vi "Show ADC Readings.vi"() -> ()   [LabVIEW 2012]
uses:
  Type/_RT Command.ctl
  Type/_RT Configuration 2.ctl
  <vilib>/Utility/config.llb/Read Key (I32).vi
  <vilib>/Utility/config.llb/Read Key (String).vi
  Configuration/_Global Configuration.vi
  <vilib>/Utility/config.llb/Write Key (I32).vi
  <vilib>/Utility/config.llb/Write Key (String).vi
  <vilib>/Utility/config.llb/NI_LVConfig.lvlib
panel:
  in  "Export":bool
  in  "Import":bool
  in  "Reserved":sgl=1.0
  in  "Tolerance":sgl
  out "Bit Pattern":i16 format="%012b"
  in  "Read":bool
  in  "Slope":sgl=1.0
  in  "Offset":sgl
  in  "Channel Name":string="Q1-ADC1-1"
  in  "Listbox":i32(listbox)
  # "(MSB)"
  # "(Enter a new value to make changes to the current row)"
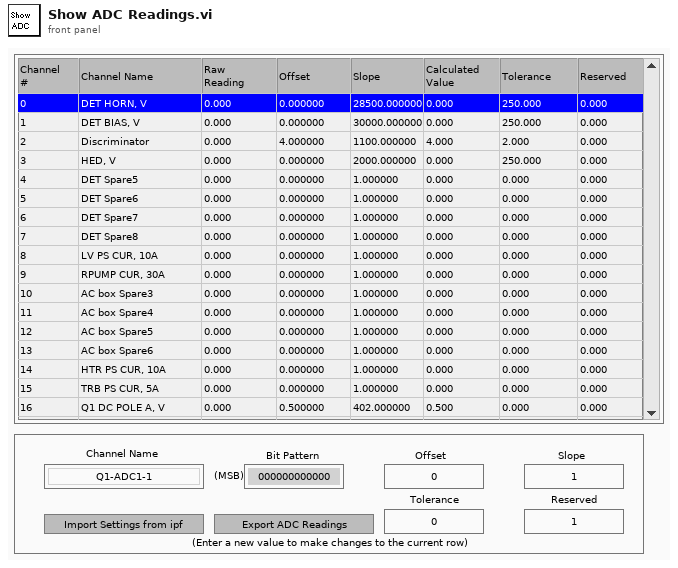
[diagram p1: front panel]
types:
  T1 = typedef "_RT Command.ctl" = enum16{"Start", "Stop", "Runtime Update", "Get Data", "Get Info", "Get Status", "Get Param", "Get Config", "Get Table", "Read ADC", "Set Oscillator", "Update Config", "Update Table", "Set All Pol", "Set Pol and DC", "Set Max Mass", "Toggle RP", "Toggle EL", "Set PIC", "Initialize Turbo", "Send Turbo Comm", "Close Turbo", "P1", "P2", "P3", "Send Serial", "Set LC Out", "Get LC In", "Read VAC", "Test Table", "Toggle Power", "Get Startup", "Set Startup", "Get ADC Table", "Set ADC Table", "Get Brief Status", "Get Detail Status", "Auxiliary Update", "Set CC Logics", "Set CC Input Logics", "Ignore Error"}
  T2 = enum32{"existing file", "new file", "new or existing file", "existing dir", "new dir", "new or existing dir", "existing file (use LLBs)", "new file (use LLBs)", "new or existing file (use LLBs)", "new or existing file or directory (use LLBs)"}
  T3 = typedef "_RT Configuration 2.ctl" = cluster{"Name":string, "Ch#":u8, "Min":dbl, "Max":dbl, "Def+":dbl, "Def-":dbl, "Offset":dbl, "Slope":dbl, "Type":u8, "Description":string, "SettleT":dbl}
  T4 = typedef "NI_LVConfig.lvlib/Config Data RefNum.ctl" = refnum<k1>
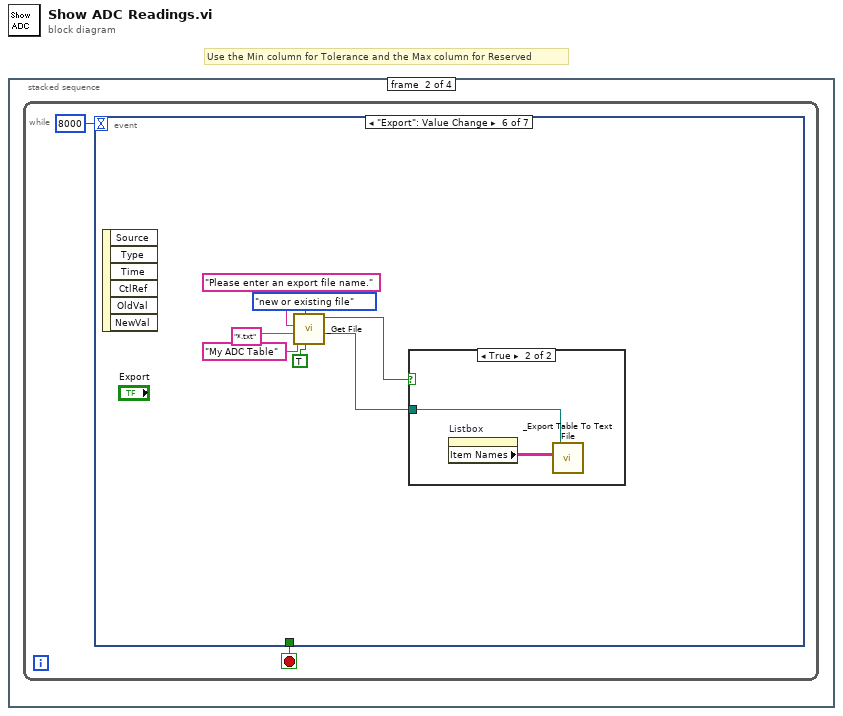
[diagram p0: block diagram]
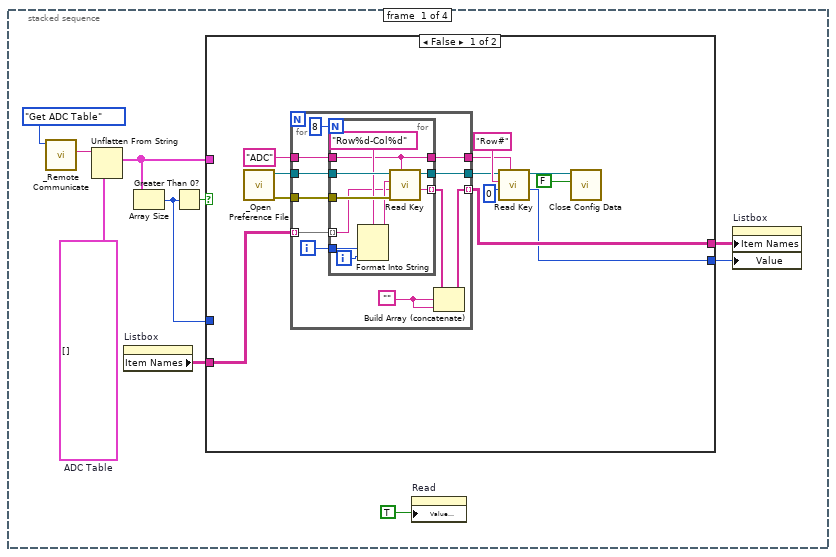
[diagram p2: hidden frame]
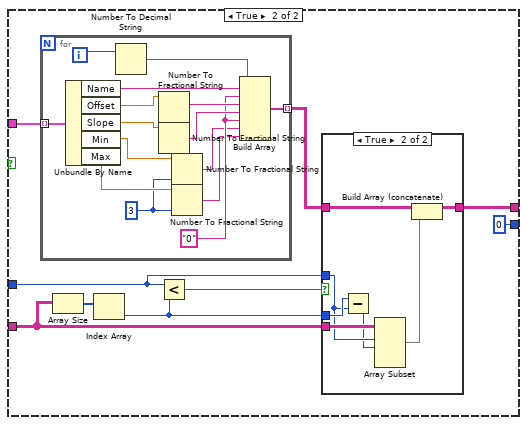
[diagram p3: hidden frame]
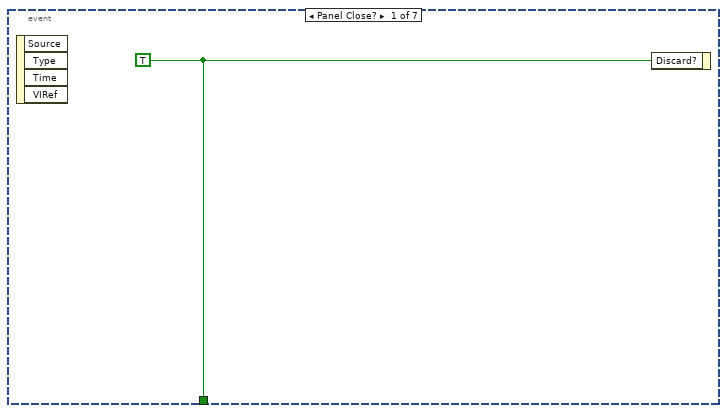
[diagram p5: hidden frame]
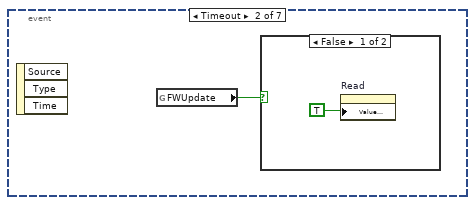
[diagram p6: hidden frame]
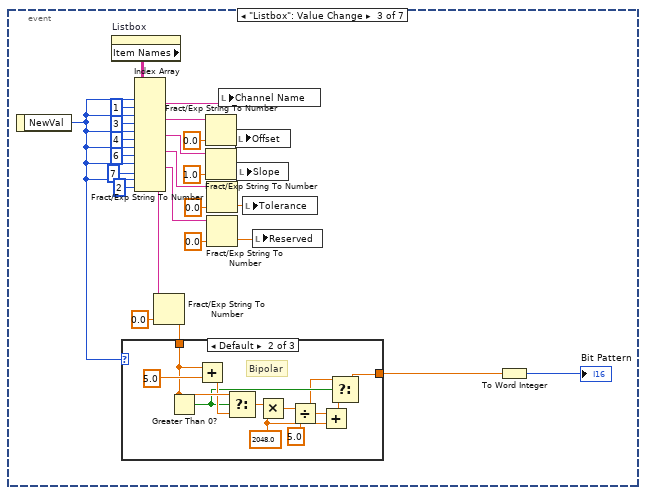
[diagram p8: hidden frame]
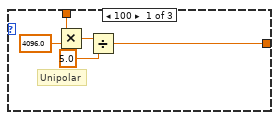
[diagram p9: hidden frame]
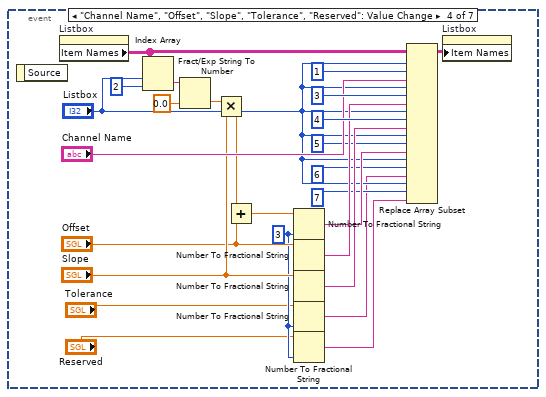
[diagram p11: hidden frame]
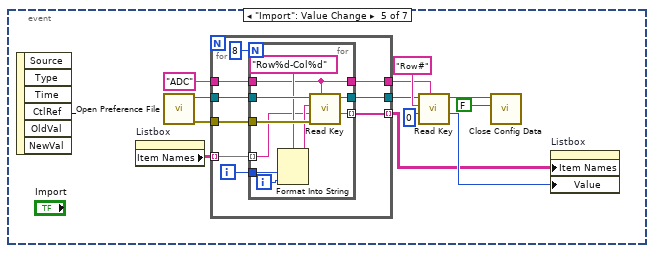
[diagram p12: hidden frame]
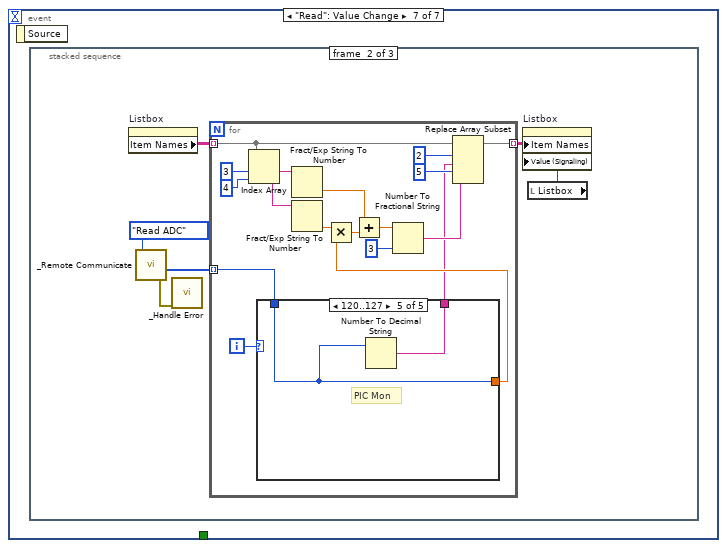
[diagram p14: hidden frame]
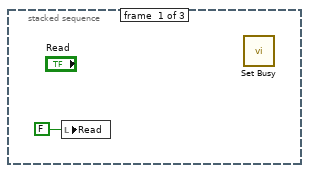
[diagram p15: hidden frame]
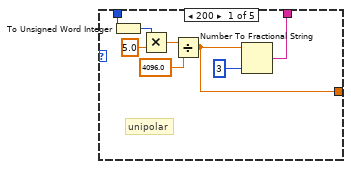
[diagram p16: hidden frame]
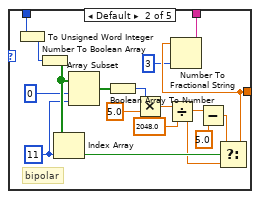
[diagram p17: hidden frame]
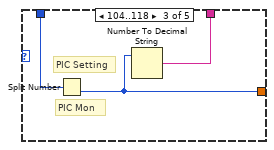
[diagram p18: hidden frame]
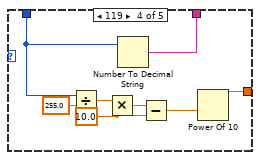
[diagram p19: hidden frame]
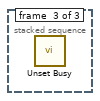
[diagram p20: hidden frame]
diagram:
  # "Use the Min column for Tolerance and the Max column for Reserved"
  n1 = stacked-sequence {
    frame #0 {
      w3 = T3[] []  # ADC Table
      n2 = call "_Remote Communicate.vi"("Command"=_RT_Command."Get ADC Table") -> ("Info"=w6:string)  [unwired: 5 in, 3 out]
      n3 = Unflatten From String(type=w3, binary string=w6) -> (value=w4:T3[])  [unwired: 1 in, 4 out]
      n4 = property on="Listbox" class="MCListbox (strict)"() -> ("Item Names"=w2:string[][])  [unwired: 2 in, 2 out]
      n5 = Array Size(array=w4) -> (size(s)=w1:i32)
      n6 = Greater Than 0?(x=w1) -> (x > 0?=w5:bool)
      n7 = case shown="False" w5 {
        tunnel: [w17 w45] -> w9
        tunnel: [w12 0 ("value")] -> w8
        tunnel: w4 -> [_ w51]
        tunnel: w2 -> [w11 w50]
        tunnel: w1 -> [_ w47]
        frame False {
          n8 = call "_Open Preference File.vi"() -> ("error"=w15:errorcluster, "refnum"=w16:T4)  [unwired: 1 in, 5 out]
          n9 = for {
            tunnel: w16 -> [w33]
            tunnel: w15 -> [w32]
            tunnel: "ADC" ("section") -> [w31]
            tunnel: [w29] -> w18
            tunnel: w11 -> [w27] mode=indexing
            tunnel: [w23] -> w17 mode=indexing
            tunnel: [w26] -> w19
            i -> [w28]
            w25 = ""
            n10 = for {
              N: 8 -> [_]
              tunnel: w33 -> [w43]
              tunnel: w32 -> [w42]
              tunnel: w31 -> [w34]
              tunnel: [w41] -> w29
              tunnel: w28 -> [w39]
              tunnel: w27 -> [w36] mode=indexing
              tunnel: [w35] -> w24 mode=indexing
              tunnel: [w34] -> w26
              i -> [w40]
              n11 = Format Into String(format string="Row%d-Col%d" ("section"), w39, w40) -> (resulting string=w37:string)  [unwired: 2 in, 1 out]
              n12 = call-poly <vilib>:"Read Key.vi"("section"=w34, "error in (no error)"=w42, "default value"=w36, "key"=w37, "refnum"=w43) -> ("value"=w35:string, "refnum out"=w41:T4)  [unwired: 1 in, 4 out]
            }
            n13 = Build Array (concatenate)(w24, w25, w25) -> (w23:string[])
          }
          n14 = call-poly <vilib>:"Read Key.vi"("section"=w19, "default value"=0 ("Listbox"), "key"="Row#" ("section"), "refnum"=w18) -> ("value"=w12:i32, "refnum out"=w21:T4)  [unwired: 1 in, 5 out]
          n15 = call <vilib>:"Close Config Data.vi"("write file if changed (T)"=FALSE ("write configuration file? (T)"), "refnum"=w21) -> ()  [unwired: 1 in, 9 out]
        }
        frame True {
          n16 = for {
            tunnel: w51 -> [w75] mode=indexing
            tunnel: [w61] -> w44 mode=indexing
            i -> [w74]
            w64 = "0"
            w69 = i16 3 ("precision (6)")
            n17 = Unbundle By Name(w75) -> ("Name"=w67:string, "Offset"=w73:dbl, "Slope"=w72:dbl, "Min"=w71:dbl, "Max"=w70:dbl)
            n18 = Number To Decimal String(number=w74) -> (decimal integer string=w68:string)  [unwired: 1 out]
            n19 = Number To Fractional String(number=w73) -> (F-format string=w66:string)  [unwired: 3 out]
            n20 = Number To Fractional String(number=w72) -> (F-format string=w65:string)  [unwired: 3 out]
            n21 = Number To Fractional String(number=w71, precision (6)=w69) -> (F-format string=w63:string)  [unwired: 2 out]
            n22 = Number To Fractional String(number=w70, precision (6)=w69) -> (F-format string=w62:string)  [unwired: 2 out]
            n23 = Build Array(w68, w67, w64, w66, w65, w64, w63, w62) -> (w61:string[])
          }
          n24 = Array Size(array=w50) -> (size(s)=w49:i32[])
          n25 = Index Array(array=w49) -> (element=w46:i32)  [unwired: 1 in]
          n26 = Less?(x=w47, y=w46) -> (x < y?=w48:bool)
          n27 = case shown="True" w48 {
            tunnel: w50 -> [_ w59]
            tunnel: w47 -> [_ w58]
            tunnel: w46 -> [_ w60]
            tunnel: w44 -> [w53 w56]
            tunnel: [w53 w55] -> w45
            frame False {
            }
            frame True {
              n28 = Subtract(x=w60, y=w58) -> (x-y=w57:i32)
              n29 = Array Subset(array=w59, index (row)=w58, length (row)=w57) -> (w54:string[][])  [unwired: 2 in]
              n30 = Build Array (concatenate)(w56, w54) -> (w55:string[][])
            }
          }
        }
      }
      n31 = property on="Read" class="Bool (strict)"("Value (Signaling)"=TRUE) -> ()  [unwired: 2 in, 2 out]
      n32 = property on="Listbox" class="MCListbox (strict)"("Item Names"=w9, "Value"=w8) -> ()  [unwired: 2 in, 2 out]
    }
    frame #1 {
      n33 = while {
        stop <- w77 stop-if-true
        n34 = event shown="[5] \"Export\": Value Change" {
          selector: _ -> [_ _ _ _ _ _ _]
          dyn-events: _ -> [_ _ _ _ _ _ _]
          timeout: 8000 -> [_ _ _ _ _ _ _]
          tunnel: [w78 _ _ _ _ _ _] -> w77
          event Panel Close? {
            w78 = TRUE ("Discard?")
            n35 = event-data() -> ()  [unwired: 5 out]
            n36 = event-data("Discard?"=w78) -> ()  [unwired: 1 in, 1 out]
          }
          event Timeout {
            n37 = event-data() -> ()  [unwired: 4 out]
            n38 = global read "_Global Configuration.vi" "FWUpdate"() -> (w79:bool)
            n39 = case shown="False" w79 {
              frame False {
                n40 = property on="Read" class="Bool (strict)"("Value (Signaling)"=TRUE) -> ()  [unwired: 2 in, 2 out]
              }
              frame True {
              }
            }
          }
          event "Listbox": Value Change {
            n41 = event-data() -> ("NewVal"=w89:i32)  [unwired: 1 out]
            n42 = property on="Listbox" class="MCListbox (strict)"() -> ("Item Names"=w106:string[][])  [unwired: 2 in, 2 out]
            n43 = Index Array(array=w106, index (row) #1=w89, index (col) #1=1 ("disabled index (col)"), index (row) #2=w89, index (col) #2=3 ("disabled index (col)"), index (row) #3=w89, index (col) #3=4 ("disabled index (col)"), index (row) #4=w89, index (col) #4=6 ("disabled index (col)"), index (row) #5=w89, index (col) #5=7 ("disabled index (col)"), index (row) #6=w89, index (col) #6=2 ("index (col)")) -> (element #1=w100:string, element #2=w102:string, element #3=w101:string, element #4=w83:string, element #5=w82:string, element #6=w81:string)
            n44 = Fract/Exp String To Number(string=w81, default (0 dbl)=sgl 0.0 ("default (0 DBL)")) -> (number=w93:sgl)  [unwired: 3 out]
            n45 = case shown="Default" w89 {
              tunnel: w93 -> [w111 w119 w123]
              tunnel: [w107 w113 w123] -> w92
              frame 100 {
                # "Unipolar"
                n46 = Multiply(x=w111, y=sgl 4096.0) -> (x*y=w109:sgl)
                n47 = Divide(x=w109, y=sgl 5.0) -> (x/y=w107:sgl)
              }
              frame Default {
                w112 = sgl 2048.0 ("y")
                # "Bipolar"
                n48 = Greater Than 0?(x=w119) -> (x > 0?=w116:bool)
                n49 = Add(x=w119, y=sgl 5.0) -> (x+y=w118:sgl)
                n50 = Select(t=w119, s=w116, f=w118) -> (s? t:f=w117:sgl)
                n51 = Multiply(x=w117, y=w112) -> (x*y=w122:sgl)
                n52 = Divide(x=w122, y=sgl 5.0) -> (x/y=w115:sgl)
                n53 = Add(x=w115, y=w112) -> (x+y=w114:sgl)
                n54 = Select(t=w115, s=w116, f=w114) -> (s? t:f=w113:sgl)
              }
              frame 104..127 {
              }
            }
            n55 = Fract/Exp String To Number(string=w102, default (0 dbl)=sgl 0.0 ("default (0 DBL)")) -> (number=w99:sgl)  [unwired: 3 out]
            n56 = Fract/Exp String To Number(string=w101, default (0 dbl)=sgl 1.0 ("default (0 DBL)")) -> (number=w97:sgl)  [unwired: 3 out]
            n57 = Fract/Exp String To Number(string=w83, default (0 dbl)=sgl 0.0 ("default (0 DBL)")) -> (number=w84:sgl)  [unwired: 3 out]
            n58 = Fract/Exp String To Number(string=w82, default (0 dbl)=sgl 0.0 ("default (0 DBL)")) -> (number=w86:sgl)  [unwired: 3 out]
            n59 = local write "Channel Name"(w100) -> ()
            n60 = local write "Offset"(w99) -> ()
            n61 = local write "Slope"(w97) -> ()
            n62 = local write "Tolerance"(w84) -> ()
            n63 = local write "Reserved"(w86) -> ()
            n64 = To Word Integer(number=w92) -> (16bit integer=→"Bit Pattern":i16)
          }
          event "Channel Name", "Offset", "Slope", "Tolerance", "Reserved": Value Change {
            w131 = i16 3 ("precision (6)")
            n65 = event-data() -> ()  [unwired: 2 out]
            n66 = property on="Listbox" class="MCListbox (strict)"() -> ("Item Names"=w141:string[][])  [unwired: 2 in, 2 out]
            n67 = Index Array(array=w141, index (row)="Listbox", index (col)=2 ("disabled index (col)")) -> (element=w139:string)
            n68 = Fract/Exp String To Number(string=w139, default (0 dbl)=sgl 0.0 ("default (0 DBL)")) -> (number=w137:sgl)  [unwired: 3 out]
            n69 = Multiply(x=w137, y="Slope") -> (x*y=w135:sgl)
            n70 = Add(x=w135, y="Offset") -> (x+y=w133:sgl)
            n71 = Number To Fractional String(number=w133, precision (6)=w131) -> (F-format string=w132:string)  [unwired: 2 out]
            n72 = Number To Fractional String(number="Offset") -> (F-format string=w144:string)  [unwired: 3 out]
            n73 = Number To Fractional String(number="Slope") -> (F-format string=w143:string)  [unwired: 3 out]
            n74 = Number To Fractional String(number="Tolerance", precision (6)=w131) -> (F-format string=w125:string)  [unwired: 2 out]
            n75 = Number To Fractional String(number="Reserved", precision (6)=w131) -> (F-format string=w124:string)  [unwired: 2 out]
            n76 = Replace Array Subset(array=w141, new element #1="Channel Name", index (row) #1="Listbox", index (col) #1=1 ("disabled index (col)"), new element #2=w144, index (row) #2="Listbox", index (col) #2=3 ("disabled index (col)"), new element #3=w143, index (row) #3="Listbox", index (col) #3=4 ("disabled index (col)"), new element #4=w132, index (row) #4="Listbox", index (col) #4=5 ("disabled index (col)"), new element #5=w125, index (row) #5="Listbox", index (col) #5=6 ("disabled index (col)"), new element #6=w124, index (row) #6="Listbox", index (col) #6=7 ("disabled index (col)")) -> (w146:string[][])
            n77 = property on="Listbox" class="MCListbox (strict)"("Item Names"=w146) -> ()  [unwired: 2 in, 2 out]
          }
          event "Import": Value Change {
            n78 = event-data() -> ()  [unwired: 7 out]
            n79 = property on="Listbox" class="MCListbox (strict)"() -> ("Item Names"=w151:string[][])  [unwired: 2 in, 2 out]
            n80 = call "_Open Preference File.vi"() -> ("error"=w153:errorcluster, "refnum"=w154:T4)  [unwired: 1 in, 5 out]
            n81 = for {
              tunnel: w154 -> [w170]
              tunnel: w153 -> [w169]
              tunnel: "ADC" ("section") -> [w168]
              tunnel: [w166] -> w155
              tunnel: w151 -> [w163] mode=indexing
              tunnel: [w162] -> w160 mode=indexing
              tunnel: [w164] -> w156
              i -> [w165]
              n82 = for {
                N: 8 -> [_]
                tunnel: w170 -> [w180]
                tunnel: w169 -> [w179]
                tunnel: w168 -> [w171]
                tunnel: [w178] -> w166
                tunnel: w165 -> [w176]
                tunnel: w163 -> [w173] mode=indexing
                tunnel: [w172] -> w162 mode=indexing
                tunnel: [w171] -> w164
                i -> [w177]
                n83 = Format Into String(format string="Row%d-Col%d" ("section"), w176, w177) -> (resulting string=w174:string)  [unwired: 2 in, 1 out]
                n84 = call-poly <vilib>:"Read Key.vi"("section"=w171, "error in (no error)"=w179, "default value"=w173, "key"=w174, "refnum"=w180) -> ("value"=w172:string, "refnum out"=w178:T4)  [unwired: 1 in, 4 out]
              }
            }
            n85 = call-poly <vilib>:"Read Key.vi"("section"=w156, "default value"=0 ("Listbox"), "key"="Row#" ("section"), "refnum"=w155) -> ("value"=w161:i32, "refnum out"=w158:T4)  [unwired: 1 in, 5 out]
            n86 = call <vilib>:"Close Config Data.vi"("write file if changed (T)"=FALSE ("write configuration file? (T)"), "refnum"=w158) -> ()  [unwired: 1 in, 9 out]
            n87 = property on="Listbox" class="MCListbox (strict)"("Item Names"=w160, "Value"=w161) -> ()  [unwired: 2 in, 2 out]
          }
          event "Export": Value Change {
            n88 = event-data() -> ()  [unwired: 7 out]
            n89 = call "_Get File.vi"("For Write (T)"=TRUE, "select mode (new or existing)"=T2."new or existing file", "default name"="My ADC Table", "extension (isd)"="*.txt" ("pattern (all files)"), "prompt"="Please enter an export file name.") -> ("Seleted File"=w181:path, "Succeeded"=w182:bool)  [unwired: 1 in, 2 out]
            n90 = case shown="True" w182 {
              tunnel: w181 -> [_ w188]
              frame False {
              }
              frame True {
                n91 = property on="Listbox" class="MCListbox (strict)"() -> ("Item Names"=w189:string[][])  [unwired: 2 in, 2 out]
                n92 = call "_Export Table To Text File.vi"("2D data"=w189, "file path (dialog if empty)"=w188) -> ()  [unwired: 4 in, 3 out]
              }
            }
          }
          event "Read": Value Change {
            n93 = event-data() -> ()  [unwired: 2 out]
            n94 = stacked-sequence {
              frame #0 {
                n95 = local write "Read"(FALSE ("Undo")) -> ()
                n96 = call <vilib>:"Set Busy.vi"() -> ()  [unwired: 4 in, 8 out]
              }
              frame #1 {
                n97 = property on="Listbox" class="MCListbox (strict)"() -> ("Item Names"=w194:string[][])  [unwired: 2 in, 2 out]
                n98 = call "_Remote Communicate.vi"("Command"=_RT_Command."Read ADC") -> ("error out"=w192:errorcluster, "Data Array"=w191:i32[])  [unwired: 5 in, 2 out]
                n99 = call "_Handle Error.vi"("error in (no error)"=w192) -> ()  [unwired: 2 in, 5 out]
                n100 = for {
                  tunnel: [w203] -> w196 mode=indexing
                  tunnel: w191 -> [w198] mode=indexing
                  tunnel: w194 -> [w202] mode=indexing
                  i -> [w201]
                  n101 = Index Array(array=w202, index #1=3 ("index"), index #2=4 ("index")) -> (element #1=w212:string, element #2=w211:string)
                  n102 = case shown="120..127" w201 {
                    tunnel: [w218 w225 w240 w243 w251] -> w200
                    tunnel: w198 -> [w216 w228 w242 w244 w251]
                    tunnel: [w217 w223 w241 w245 w252] -> w197
                    frame 200 {
                      # "unipolar"
                      n103 = To Unsigned Word Integer(number=w216) -> (unsigned 16bit integer=w215:u16)
                      n104 = Multiply(x=w215, y=sgl 5.0) -> (x*y=w221:sgl)
                      n105 = Divide(x=w221, y=sgl 4096.0) -> (x/y=w218:sgl)
                      n106 = Number To Fractional String(number=w218, precision (6)=i16 3) -> (F-format string=w217:string)  [unwired: 2 out]
                    }
                    frame Default {
                      w237 = 11 ("index")
                      # "bipolar"
                      n107 = To Unsigned Word Integer(number=w228) -> (unsigned 16bit integer=w227:u16)
                      n108 = Number To Boolean Array(number=w227) -> (Boolean array=w239:bool[])
                      n109 = Index Array(array=w239, index=w237) -> (element=w232:bool)
                      n110 = Array Subset(array=w239, index=0, length=w237) -> (w236:bool[])
                      n111 = Boolean Array To Number(Boolean array=w236) -> (number=w233:u32)
                      n112 = Multiply(x=w233, y=sgl 5.0) -> (x*y=w226:sgl)
                      n113 = Divide(x=w226, y=sgl 2048.0) -> (x/y=w231:sgl)
                      n114 = Subtract(x=w231, y=sgl 5.0) -> (x-y=w229:sgl)
                      n115 = Select(t=w229, s=w232, f=w231) -> (s? t:f=w225:sgl)
                      n116 = Number To Fractional String(number=w225, precision (6)=i16 3) -> (F-format string=w223:string)  [unwired: 2 out]
                    }
                    frame 104..118 {
                      # "PIC Setting"
                      # "PIC Mon"
                      n117 = Split Number(x=w242) -> (lo(x)=w240:u16)  [unwired: 1 out]
                      n118 = Number To Decimal String(number=w240) -> (decimal integer string=w241:string)  [unwired: 1 out]
                    }
                    frame 119 {
                      w246 = sgl 10.0 ("y")
                      n119 = Divide(x=w244, y=sgl 255.0) -> (x/y=w249:sgl)
                      n120 = Multiply(x=w249, y=w246) -> (x*y=w248:sgl)
                      n121 = Number To Decimal String(number=w244) -> (decimal integer string=w245:string)  [unwired: 1 out]
                      n122 = Subtract(x=w248, y=w246) -> (x-y=w247:sgl)
                      n123 = Power Of 10(x=w247) -> (10^x=w243:sgl)
                    }
                    frame 120..127 {
                      # "PIC Mon"
                      n124 = Number To Decimal String(number=w251) -> (decimal integer string=w252:string)  [unwired: 1 out]
                    }
                  }
                  n125 = Fract/Exp String To Number(string=w212) -> (number=w208:dbl)  [unwired: 4 out]
                  n126 = Fract/Exp String To Number(string=w211) -> (number=w210:dbl)  [unwired: 4 out]
                  n127 = Multiply(x=w210, y=w200) -> (x*y=w209:dbl)
                  n128 = Add(x=w208, y=w209) -> (x+y=w207:dbl)
                  n129 = Number To Fractional String(number=w207, precision (6)=i16 3) -> (F-format string=w199:string)  [unwired: 2 out]
                  n130 = Replace Array Subset(array=w202, new element #1=w197, index #1=2 ("index"), new element #2=w199, index #2=5 ("index")) -> (w203:string[])
                }
                n131 = local read "Listbox"() -> (w195:i32)
                n132 = property on="Listbox" class="MCListbox (strict)"("Item Names"=w196, "Value (Signaling)"=w195) -> ()  [unwired: 2 in, 2 out]
              }
              frame #2 {
                n133 = call <vilib>:"Unset Busy.vi"() -> ()  [unwired: 2 in, 10 out]
              }
            }
          }
        }
      }
    }
    frame #2 {
      n134 = property on="Listbox" class="MCListbox (strict)"() -> ("Item Names"=w257:string[][])  [unwired: 2 in, 2 out]
      n135 = call "_Open Preference File.vi"() -> ("error"=w266:errorcluster, "refnum"=w267:T4)  [unwired: 1 in, 5 out]
      n136 = for {
        tunnel: w267 -> [w288]
        tunnel: "ADC" ("section") -> [w286]
        tunnel: [w284] -> w264
        tunnel: w257 -> [w282] mode=indexing
        tunnel: [w281] -> w262
        shift-right: [w280] -> w259
        shift-left: w266 -> [w287]
        i -> [w283]
        n137 = for {
          N: 8 -> [_]
          tunnel: w288 -> [w298]
          tunnel: w286 -> [w290]
          tunnel: [w296] -> w284
          tunnel: w283 -> [w294]
          tunnel: w282 -> [w291] mode=indexing
          tunnel: [w290] -> w281
          shift-right: [w289] -> w280
          shift-left: w287 -> [w297]
          i -> [w295]
          n138 = Format Into String(format string="Row%d-Col%d" ("section"), w294, w295) -> (resulting string=w292:string)  [unwired: 2 in, 1 out]
          n139 = call-poly <vilib>:"Write Key.vi"("section"=w290, "error in (no error)"=w297, "value"=w291, "key"=w292, "refnum"=w298) -> ("error out"=w289:errorcluster, "refnum out"=w296:T4)  [unwired: 1 in, 4 out]
        }
      }
      n140 = for {
        tunnel: w257 -> [w279] mode=indexing
        tunnel: T3 {"Name"="", "Ch#"=0, "Min"=0.0, "Max"=0.0, "Def+"=0.0, "Def-"=0.0, "Offset"=0.0, "Slope"=0.0, "Type"=0, "Description"="", "SettleT"=0.0} ("Configuration") -> [w274]
        tunnel: [w268] -> w253 mode=indexing
        n141 = Index Array(array=w279) -> (element #2=w273:string, element #4=w278:string, element #5=w277:string, element #7=w276:string, element #8=w275:string)  [unwired: 8 in, 3 out]
        n142 = Fract/Exp String To Number(string=w278) -> (number=w272:dbl)  [unwired: 4 out]
        n143 = Fract/Exp String To Number(string=w277) -> (number=w271:dbl)  [unwired: 4 out]
        n144 = Fract/Exp String To Number(string=w276) -> (number=w270:dbl)  [unwired: 4 out]
        n145 = Fract/Exp String To Number(string=w275) -> (number=w269:dbl)  [unwired: 4 out]
        n146 = Bundle By Name(cluster=w274, "Name"=w273, "Offset"=w272, "Slope"=w271, "Min"=w270, "Max"=w269) -> (w268:T3)
      }
      n147 = local read "Listbox"() -> (w260:i32)
      n148 = call-poly <vilib>:"Write Key.vi"("section"=w262, "error in (no error)"=w259, "value"=w260, "key"="Row#" ("section"), "refnum"=w264) -> ("error out"=w258:errorcluster, "refnum out"=w263:T4)  [unwired: 5 out]
      n149 = Flatten To String(anything=w253) -> (data string=w254:string)  [unwired: 1 in, 4 out]
      n150 = call <vilib>:"Close Config Data.vi"("error in (no error)"=w258, "refnum"=w263) -> ()  [unwired: 1 in, 9 out]
      n151 = call "_Remote Communicate.vi"("String"=w254, "Command"=_RT_Command."Set ADC Table") -> ()  [unwired: 4 in, 4 out]
    }
    frame #3 {
      n152 = property class="VI"("Front Panel.Open"=FALSE ("Front Panel Window:Open")) -> ()  [unwired: 2 in, 2 out]
    }
  }
